vi "BundledShapeCache.vi"(8 "error in (no error)":errorcluster, 11 "BundledShapeCache in":refnum<class "BundledShapeCache.lvclass">) -> (0 "error out":errorcluster, 3 "BundledShapeCache out":refnum<class "BundledShapeCache.lvclass">)   [LabVIEW 2017, in "BundledShapeCache.lvclass"]
uses:
  BundledShapeCache.lvclass
  Circle Class/pCircle.lvclass
  C:/Users/fflores/Documents/LabVIEW-Open-Projects/LabIVEW OOP Design Patterns/Prototype Pattern/Shape Class/pShape.lvclass
  Rectangle Class/pRectangle.lvclass
  Rectangle Class/pRectangle.lvclass/pRectangle.ctl
  Circle Class/pCircle.lvclass/pCircle.ctl
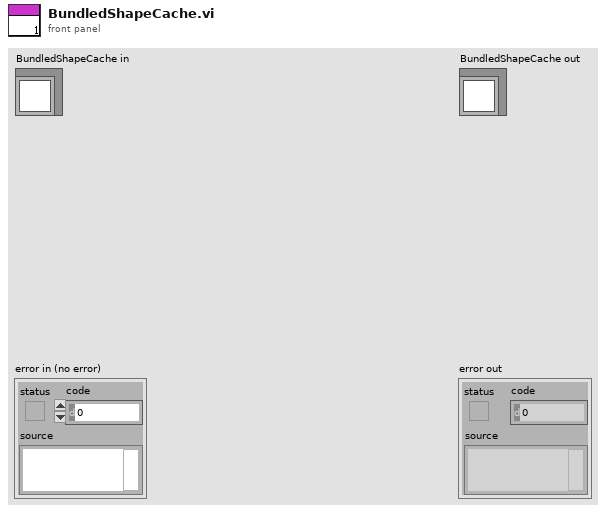
[diagram p1: front panel]
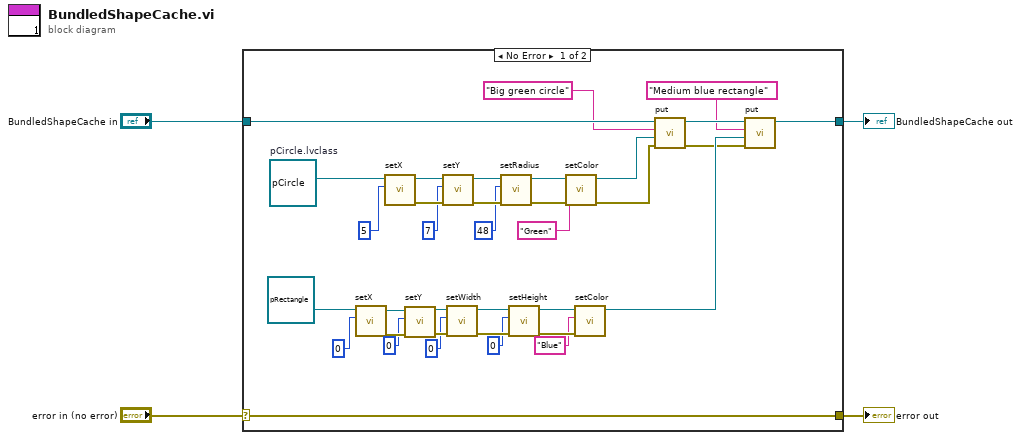
[diagram p0: block diagram]
diagram:
  n1 = case shown="No Error" "error in (no error)" {
    selector: "error in (no error)" -> [w38 w41]
    tunnel: [w38 w41] -> w3
    tunnel: [w10 w40] -> w1
    tunnel: "BundledShapeCache in" -> [w39 w40]
    frame No Error {
      w33 = refnum<class "pCircle.lvclass"> refnum  # pCircle.lvclass
      n2 = call "setX.vi"("x"=0, "pRectangle in"=refnum<class "pRectangle.lvclass"> refnum ("pRectangle.lvclass")) -> ("error out"=w25:errorcluster, "pRectangle out"=w26:refnum<class "pRectangle.lvclass">)  [unwired: 8 in]
      n3 = call "setX.vi"("x"=5, "pCircle in"=w33) -> ("error out"=w36:errorcluster, "pCircle out"=w37:refnum<class "pCircle.lvclass">)  [unwired: 8 in]
      n4 = call "setY.vi"("error in (no error)"=w25, "y"=0, "pRectangle in"=w26) -> ("error out"=w23:errorcluster, "pRectangle out"=w24:refnum<class "pRectangle.lvclass">)  [unwired: 7 in]
      n5 = call "setY.vi"("error in (no error)"=w36, "y"=7, "pCircle in"=w37) -> ("error out"=w34:errorcluster, "pCircle out"=w35:refnum<class "pCircle.lvclass">)  [unwired: 7 in]
      n6 = call "setWidth.vi"("error in (no error)"=w23, "width"=0, "pRectangle in"=w24) -> ("error out"=w21:errorcluster, "pRectangle out"=w22:refnum<class "pRectangle.lvclass">)  [unwired: 7 in]
      n7 = call "setRadius.vi"("error in (no error)"=w34, "radius"=48, "pCircle in"=w35) -> ("error out"=w28:errorcluster, "pCircle out"=w29:refnum<class "pCircle.lvclass">)  [unwired: 7 in]
      n8 = call "setHeight.vi"("error in (no error)"=w21, "height"=0, "pRectangle in"=w22) -> ("error out"=w19:errorcluster, "pRectangle out"=w20:refnum<class "pRectangle.lvclass">)  [unwired: 7 in]
      n9 = call "setColor.vi"("error in (no error)"=w28, "color"="Green", "pCircle in"=w29) -> ("error out"=w6:errorcluster, "pCircle out"=w11:refnum<class "pCircle.lvclass">)  [unwired: 7 in]
      n10 = call "setColor.vi"("error in (no error)"=w19, "color"="Blue", "pRectangle in"=w20) -> ("pRectangle out"=w9:refnum<class "pRectangle.lvclass">)  [unwired: 7 in, 1 out]
      n11 = call "put.vi"("error in (no error)"=w6, "pShape.lvclass"=w11, "Key"="Big green circle", "BundledShapeCache in"=w39) -> ("error out"=w5:errorcluster, "BundledShapeCache out"=w12:refnum<class "BundledShapeCache.lvclass">)  [unwired: 6 in]
      n12 = call "put.vi"("error in (no error)"=w5, "pShape.lvclass"=w9, "Key"="Medium blue rectangle", "BundledShapeCache in"=w12) -> ("BundledShapeCache out"=w10:refnum<class "BundledShapeCache.lvclass">)  [unwired: 6 in, 1 out]
    }
    frame Error {
    }
  }
  "error out" <- w3
  "BundledShapeCache out" <- w1
